vi "writeToXML.vi"(8 "error in (no error)":errorcluster, 10 "ClassLabel":string, 11 "instrumentSelect in":refnum<class "InstrumentSelect.lvclass">) -> (0 "error out":errorcluster, 2 "XML out":string, 3 "instrumentSelect out":refnum<class "InstrumentSelect.lvclass">)   [LabVIEW 2022 SP3, in "TCSDataDefinitions.lvlib" / "TCSCommand.lvlib" / "InstrumentSelect.lvclass"]
uses:
  InstrumentSelect.lvclass
  InstrumentSelect.lvclass/InstrumentSelect.ctl
  TCSTcsCommand/TCSTcsCommand.lvclass
  <userlib>/Common/XML/XMLGenerator/XMLGenerator.lvclass
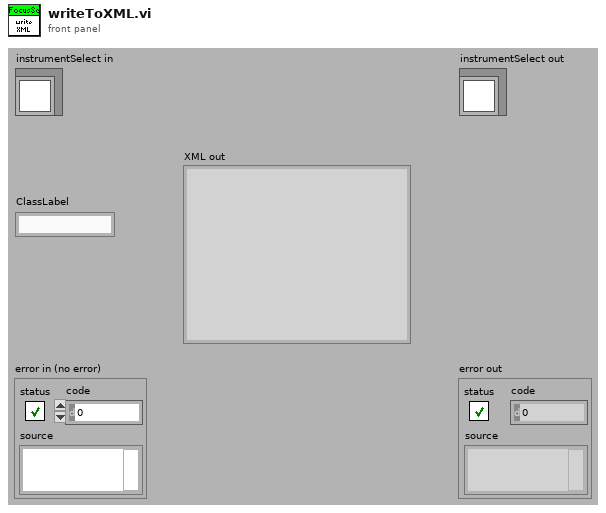
[diagram p1: front panel]
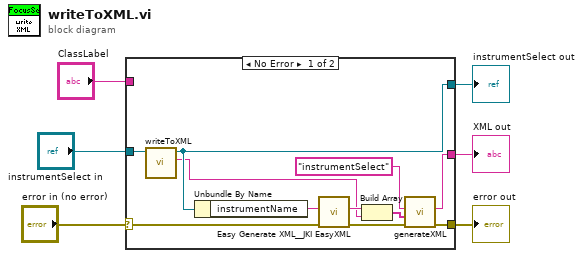
[diagram p0: block diagram]
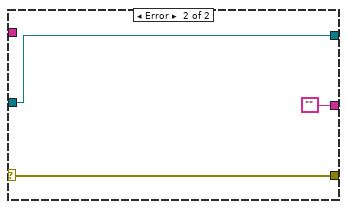
[diagram p2: hidden frame]
diagram:
  n1 = case shown="No Error" "error in (no error)" {
    selector: "error in (no error)" -> [w13 w20]
    tunnel: [w12 w20] -> w5
    tunnel: [w9 w19] -> w3
    tunnel: "instrumentSelect in" -> [w10 w19]
    tunnel: "ClassLabel" -> [_ _]
    tunnel: [w11 ""] -> w1
    frame No Error {
      n2 = call-parent "writeToXML.vi"("TCSTcsCommand in"=w10) -> ("XML out"=w8:string, "TCSTcsCommand out"=w9:refnum<class "InstrumentSelect.lvclass">)  [unwired: 8 in, 1 out]
      n3 = Unbundle By Name(w9) -> ("instrumentName"=w17:string)
      n4 = call <vilib>:"Easy Generate XML__JKI EasyXML.vi"("error in (no error)"=w13, "LabVIEW Data"=w17) -> ("error out"=w14:errorcluster, "XML String"=w16:string)  [unwired: 8 in]
      n5 = Build Array(w16, w8) -> (w15:string[])
      n6 = call <userlib>:"generateXML.vi"("error in"=w14, "childrenXML"=w15, "elementName"="instrumentSelect" ("Class Label")) -> ("error out"=w12:errorcluster, "XML out"=w11:string)  [unwired: 6 in, 1 out]
    }
    frame Error {
    }
  }
  "error out" <- w5
  "instrumentSelect out" <- w3
  "XML out" <- w1
